vi "NanonisLagTest.vi"() -> ()   [LabVIEW 2017]
panel:
  in  "stop":bool
  out "Iterations":i32
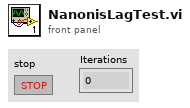
[diagram p1: front panel]
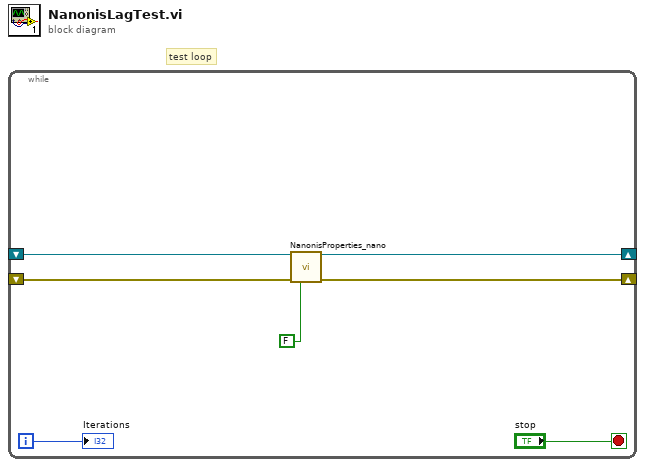
[diagram p0: block diagram]
diagram:
  # "test loop"
  n1 = while {
    shift-right: [w5] -> _
    shift-left: _ -> [w4]
    shift-right: [w6] -> _
    shift-left: _ -> [w7]
    i -> [w3]
    stop <- "stop" stop-if-true
    n2 = call "NanonisProperties_nano.vi"("Application reference"=w7, "Error in"=w4, "Z Write?"=FALSE) -> ("Application ref out"=w6:refnum<vi>, "error out"=w5:errorcluster)  [unwired: 6 in, 5 out]
    "Iterations" <- w3
  }
